vi "FGV DATA.vi"(6 "error in (no error)":errorcluster, 7 "Enum":enum16{"SET", "GET"}(ring), 8 "SET??":bool[](array[boolean]), 9 "TEMPERATURA IN":dbl, 10 "HUMEDAD IN":dbl, 11 "PH IN":dbl) -> (1 "TEMPERATURA OUT":dbl, 2 "HUMEDAD OUT":dbl, 3 "PH OUT":dbl, 4 "error out":errorcluster)   [LabVIEW 2019]
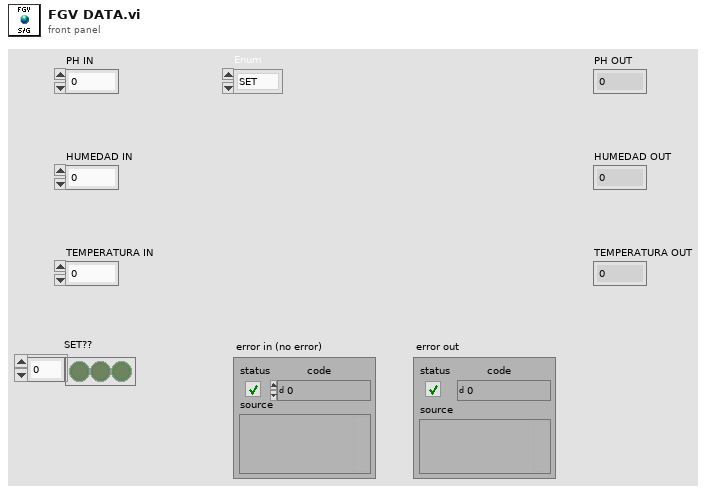
[diagram p1: front panel]
types:
  T1 = cluster{"SET??[0]":bool, "SET??[1]":bool, "SET??[2]":bool, "SET??[3]":bool, "SET??[4]":bool, "SET??[5]":bool, "SET??[6]":bool, "SET??[7]":bool, "SET??[8]":bool}
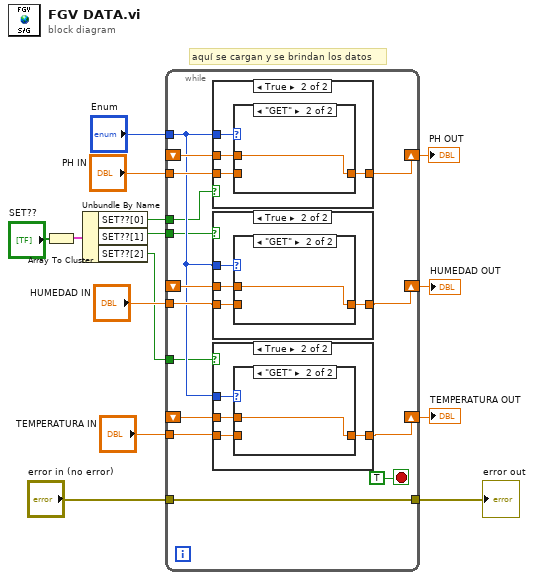
[diagram p0: block diagram]
diagram:
  # "aquí se cargan y se brindan los datos"
  n1 = Array To Cluster(array="SET??") -> (cluster=w6:T1)
  n2 = Unbundle By Name(w6) -> ("SET??[0]"=w5:bool, "SET??[1]"=w4:bool, "SET??[2]"=w3:bool)
  n3 = while {
    tunnel: "PH IN" -> [w28]
    shift-right: [w27] -> w10
    shift-left: _ -> [w26]
    tunnel: "Enum" -> [w23]
    tunnel: "HUMEDAD IN" -> [w24]
    tunnel: "TEMPERATURA IN" -> [w19]
    shift-right: [w22] -> w8
    shift-left: _ -> [w25]
    shift-right: [w21] -> w9
    shift-left: _ -> [w20]
    tunnel: w5 -> [w18]
    tunnel: w4 -> [w17]
    tunnel: w3 -> [w16]
    tunnel: "error in (no error)" -> [w15]
    tunnel: [w15] -> w1
    stop <- TRUE stop-if-true
    n4 = case shown="True" w18 {
      tunnel: w28 -> [_ w48]
      tunnel: [w44 w47] -> w27
      tunnel: w26 -> [w44 w46]
      tunnel: w23 -> [_ w45]
      frame False {
      }
      frame True {
        n5 = case shown="\"GET\"" w45 {
          tunnel: w48 -> [w49 _]
          tunnel: [w49 w50] -> w47
          tunnel: w46 -> [_ w50]
          frame "SET", Default {
          }
          frame "GET" {
          }
        }
      }
    }
    n6 = case shown="True" w17 {
      tunnel: w24 -> [_ w41]
      tunnel: [w37 w40] -> w22
      tunnel: w25 -> [w37 w39]
      tunnel: w23 -> [_ w38]
      frame False {
      }
      frame True {
        n7 = case shown="\"GET\"" w38 {
          tunnel: w41 -> [w42 _]
          tunnel: [w42 w43] -> w40
          tunnel: w39 -> [_ w43]
          frame "SET", Default {
          }
          frame "GET" {
          }
        }
      }
    }
    n8 = case shown="True" w16 {
      tunnel: w19 -> [_ w34]
      tunnel: [w30 w33] -> w21
      tunnel: w20 -> [w30 w32]
      tunnel: w23 -> [_ w31]
      frame False {
      }
      frame True {
        n9 = case shown="\"GET\"" w31 {
          tunnel: w34 -> [w35 _]
          tunnel: [w35 w36] -> w33
          tunnel: w32 -> [_ w36]
          frame "SET", Default {
          }
          frame "GET" {
          }
        }
      }
    }
  }
  "PH OUT" <- w10
  "HUMEDAD OUT" <- w8
  "TEMPERATURA OUT" <- w9
  "error out" <- w1
